vi "Handle Error.vi"(8 "error in (no error)":errorcluster, 11 "Graph in":refnum<class "Graph.lvclass">) -> (0 "error out":errorcluster, 2 "stop actor?":bool=TRUE, 3 "Graph out":refnum<class "Graph.lvclass">)   [LabVIEW 2020, in "Graph.lvlib" / "Graph.lvclass"]
doc: "(<B>Filename</B>: Actor Framework.lvlib:Actor.lvclass:Handle Error.vi)\n\nDefines how the actor handles an error that occurred while processing a message. By default, this method does nothing except stop the actor.\n\nThis implementation generates the End event if the actors is stopped."
uses:
  Graph.lvclass
  Graph.lvclass/Graph.ctl
  <vilib>/event_ctls.llb/usereventprio.ctl
  PPL/HDH.Actor Framework.Core.Actor.lvlibp/1abvi3w/vi.lib/ActorFramework/Actor/Actor.lvclass
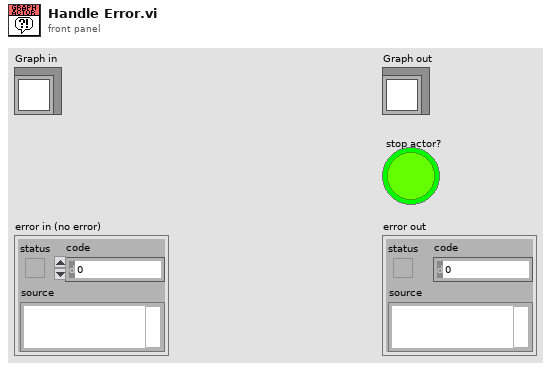
[diagram p1: front panel]
types:
  T1 = typedef "usereventprio.ctl" = enum32{"high priority", "normal priority"}
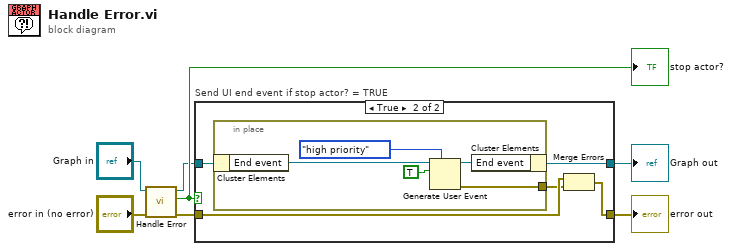
[diagram p0: block diagram]
diagram:
  n1 = call-parent "Handle Error.vi"("error in (no error)"="error in (no error)", "Actor in"="Graph in") -> ("error out"=w3:errorcluster, "stop actor?"=w5:bool, "Actor out"=w1:refnum<class "Graph.lvclass">)  [unwired: 7 in]
  "stop actor?" <- w5
  n2 = case "Send UI end event if stop actor? = TRUE" shown="True" w5 {
    tunnel: [w9 w10] -> w4
    tunnel: w3 -> [w9 w12]
    tunnel: [w8 w13] -> w2
    tunnel: w1 -> [w8 w14]
    frame False {
    }
    frame True {
      n3 = in-place {
        in-place-border: [w15] -> w11
        n4 = in-place-cluster #1(w14) -> ("End event"=w19:refnum<user-event>)
        n5 = Generate User Event(priority (normal)=usereventprio."high priority", user event=w19, event data cluster=TRUE ("event data")) -> (user event out=w16:refnum<user-event>, error out=w15:errorcluster)  [unwired: 1 in]
        n6 = in-place-cluster #1("End event"=w16) -> (w13:refnum<class "Graph.lvclass">)
      }
      n7 = Merge Errors(w12, w11) -> (w10:errorcluster)
    }
  }
  "Graph out" <- w2
  "error out" <- w4
